vi "3654GetDashValues.vi"   [LabVIEW 2017]
uses:
  <vilib>/Rock Robotics/Network Tables/NT Read Boolean.vi
  Robot Global Data.vi
  <vilib>/Rock Robotics/Network Tables/NT Read Number.vi
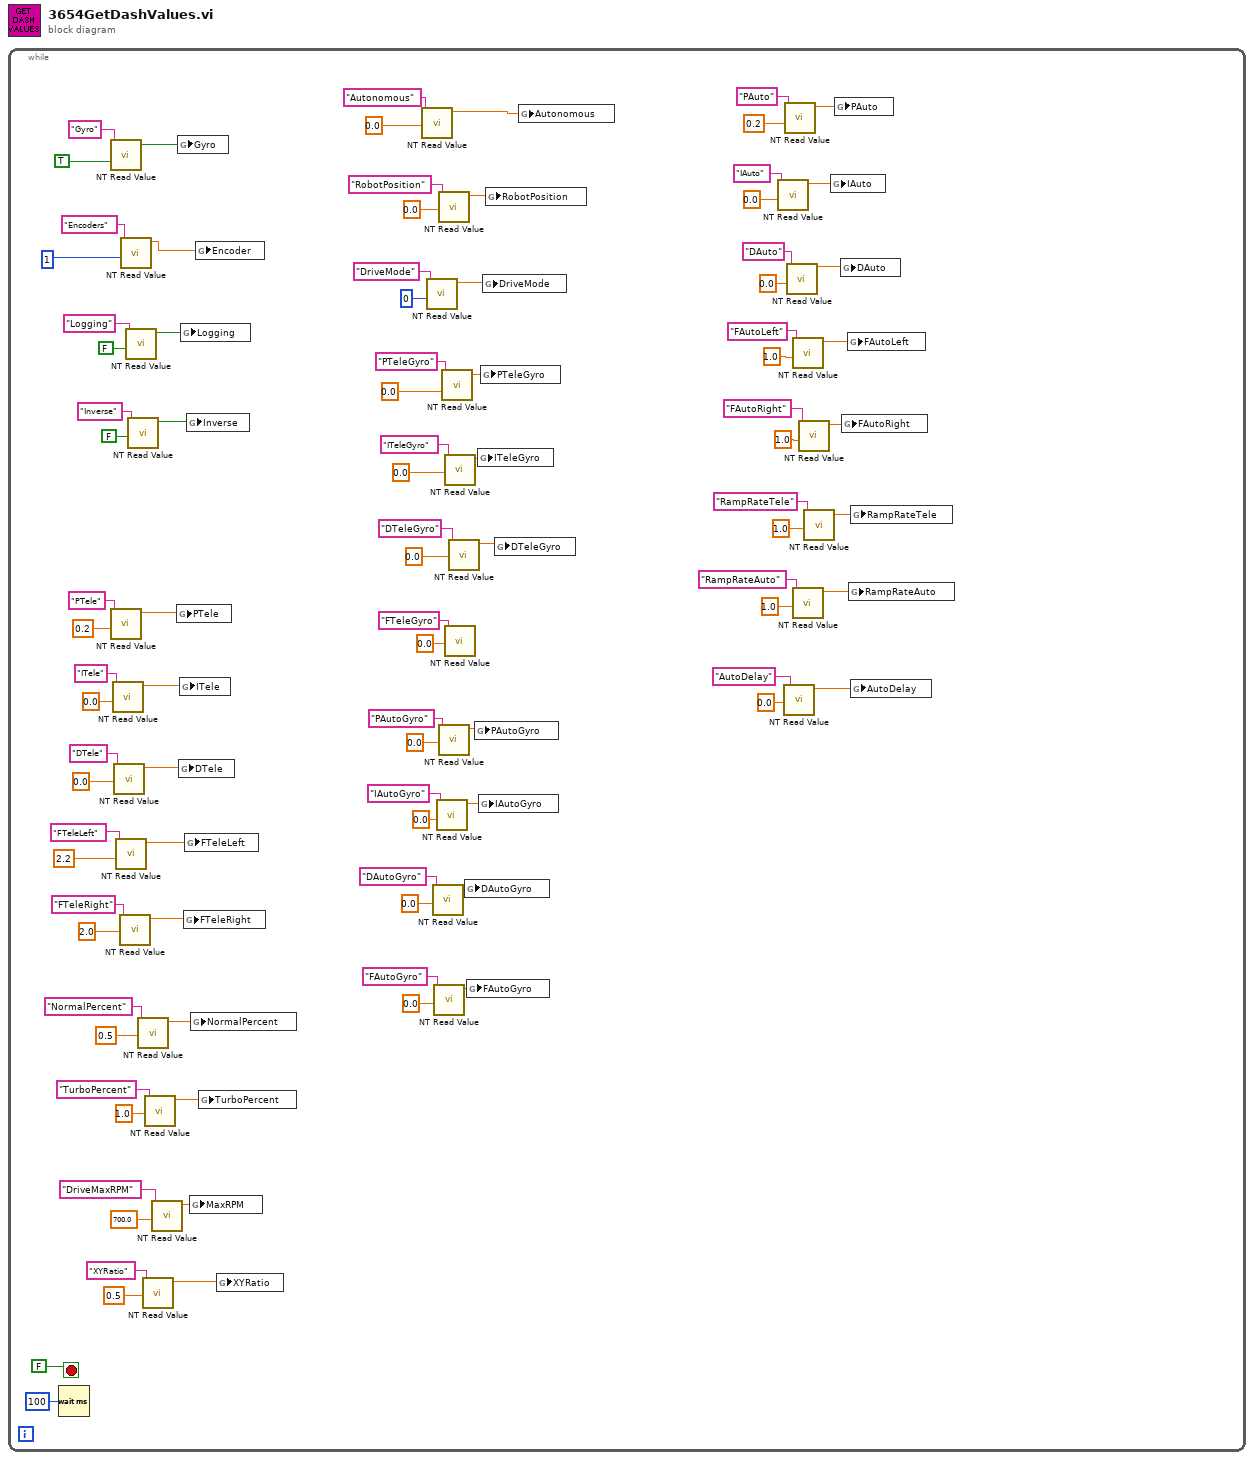
[diagram p0: block diagram]
diagram:
  n1 = while {
    stop <- FALSE stop-if-true
    n2 = Wait (ms)(milliseconds to wait=u32 100) -> ()  [unwired: 1 out]
    n3 = call-poly <vilib>:"NT Read Value.vi"("Default Value"=TRUE, "Name"="Gyro") -> ("Boolean"=w96:bool)  [unwired: 8 in, 1 out]
    n4 = call-poly <vilib>:"NT Read Value.vi"("Default Value"=0.2, "Name"="PTele") -> ("Numeric"=w79:dbl)  [unwired: 8 in, 1 out]
    n5 = call-poly <vilib>:"NT Read Value.vi"("Default Value"=0.0, "Name"="ITele") -> ("Numeric"=w80:dbl)  [unwired: 8 in, 1 out]
    n6 = call-poly <vilib>:"NT Read Value.vi"("Default Value"=0.0, "Name"="DTele") -> ("Numeric"=w81:dbl)  [unwired: 8 in, 1 out]
    n7 = call-poly <vilib>:"NT Read Value.vi"("Default Value"=2.2, "Name"="FTeleLeft") -> ("Numeric"=w72:dbl)  [unwired: 8 in, 1 out]
    n8 = call-poly <vilib>:"NT Read Value.vi"("Default Value"=2.0, "Name"="FTeleRight") -> ("Numeric"=w71:dbl)  [unwired: 8 in, 1 out]
    n9 = call-poly <vilib>:"NT Read Value.vi"("Default Value"=1, "Name"="Encoders") -> ("Numeric"=w2:dbl)  [unwired: 8 in, 1 out]
    n10 = call-poly <vilib>:"NT Read Value.vi"("Default Value"=FALSE, "Name"="Logging") -> ("Boolean"=w31:bool)  [unwired: 8 in, 1 out]
    n11 = call-poly <vilib>:"NT Read Value.vi"("Default Value"=FALSE, "Name"="Inverse") -> ("Boolean"=w32:bool)  [unwired: 8 in, 1 out]
    n12 = call-poly <vilib>:"NT Read Value.vi"("Default Value"=0.5, "Name"="NormalPercent") -> ("Numeric"=w49:dbl)  [unwired: 8 in, 1 out]
    n13 = call-poly <vilib>:"NT Read Value.vi"("Default Value"=0.5, "Name"="XYRatio") -> ("Numeric"=w8:dbl)  [unwired: 8 in, 1 out]
    n14 = call-poly <vilib>:"NT Read Value.vi"("Default Value"=1.0, "Name"="TurboPercent") -> ("Numeric"=w46:dbl)  [unwired: 8 in, 1 out]
    n15 = call-poly <vilib>:"NT Read Value.vi"("Default Value"=700.0, "Name"="DriveMaxRPM") -> ("Numeric"=w11:dbl)  [unwired: 8 in, 1 out]
    n16 = global write "Robot Global Data.vi" "PTele"(w79) -> ()
    n17 = global write "Robot Global Data.vi" "Gyro"(w96) -> ()
    n18 = global write "Robot Global Data.vi" "DTele"(w81) -> ()
    n19 = global write "Robot Global Data.vi" "ITele"(w80) -> ()
    n20 = global write "Robot Global Data.vi" "Logging"(w31) -> ()
    n21 = global write "Robot Global Data.vi" "FTeleRight"(w71) -> ()
    n22 = global write "Robot Global Data.vi" "FTeleLeft"(w72) -> ()
    n23 = global write "Robot Global Data.vi" "Inverse"(w32) -> ()
    n24 = global write "Robot Global Data.vi" "MaxRPM"(w11) -> ()
    n25 = global write "Robot Global Data.vi" "NormalPercent"(w49) -> ()
    n26 = global write "Robot Global Data.vi" "Encoder"(w2) -> ()
    n27 = global write "Robot Global Data.vi" "TurboPercent"(w46) -> ()
    n28 = global write "Robot Global Data.vi" "XYRatio"(w8) -> ()
    n29 = call-poly <vilib>:"NT Read Value.vi"("Default Value"=0.0, "Name"="Autonomous") -> ("Numeric"=w93:dbl)  [unwired: 8 in, 1 out]
    n30 = call-poly <vilib>:"NT Read Value.vi"("Default Value"=0, "Name"="DriveMode") -> ("Numeric"=w5:dbl)  [unwired: 8 in, 1 out]
    n31 = call-poly <vilib>:"NT Read Value.vi"("Default Value"=0.0, "Name"="DAutoGyro") -> ("Numeric"=w41:dbl)  [unwired: 8 in, 1 out]
    n32 = call-poly <vilib>:"NT Read Value.vi"("Default Value"=0.0, "Name"="FAutoGyro") -> ("Numeric"=w20:dbl)  [unwired: 8 in, 1 out]
    n33 = call-poly <vilib>:"NT Read Value.vi"("Default Value"=0.0, "Name"="IAutoGyro") -> ("Numeric"=w42:dbl)  [unwired: 8 in, 1 out]
    n34 = call-poly <vilib>:"NT Read Value.vi"("Default Value"=0.0, "Name"="RobotPosition") -> ("Numeric"=w26:dbl)  [unwired: 8 in, 1 out]
    n35 = call-poly <vilib>:"NT Read Value.vi"("Default Value"=0.0, "Name"="PAutoGyro") -> ("Numeric"=w43:dbl)  [unwired: 8 in, 1 out]
    n36 = call-poly <vilib>:"NT Read Value.vi"("Default Value"=0.0, "Name"="PTeleGyro") -> ("Numeric"=w88:dbl)  [unwired: 8 in, 1 out]
    n37 = call-poly <vilib>:"NT Read Value.vi"("Default Value"=0.0, "Name"="ITeleGyro") -> ("Numeric"=w86:dbl)  [unwired: 8 in, 1 out]
    n38 = call-poly <vilib>:"NT Read Value.vi"("Default Value"=0.0, "Name"="FTeleGyro") -> ()  [unwired: 8 in, 2 out]
    n39 = call-poly <vilib>:"NT Read Value.vi"("Default Value"=0.0, "Name"="DTeleGyro") -> ("Numeric"=w87:dbl)  [unwired: 8 in, 1 out]
    n40 = global write "Robot Global Data.vi" "DAutoGyro"(w41) -> ()
    n41 = global write "Robot Global Data.vi" "FAutoGyro"(w20) -> ()
    n42 = global write "Robot Global Data.vi" "PAutoGyro"(w43) -> ()
    n43 = global write "Robot Global Data.vi" "ITeleGyro"(w86) -> ()
    n44 = global write "Robot Global Data.vi" "IAutoGyro"(w42) -> ()
    n45 = global write "Robot Global Data.vi" "PTeleGyro"(w88) -> ()
    n46 = global write "Robot Global Data.vi" "DriveMode"(w5) -> ()
    n47 = global write "Robot Global Data.vi" "RobotPosition"(w26) -> ()
    n48 = global write "Robot Global Data.vi" "DTeleGyro"(w87) -> ()
    n49 = global write "Robot Global Data.vi" "Autonomous"(w93) -> ()
    n50 = call-poly <vilib>:"NT Read Value.vi"("Default Value"=0.0, "Name"="IAuto") -> ("Numeric"=w63:dbl)  [unwired: 8 in, 1 out]
    n51 = call-poly <vilib>:"NT Read Value.vi"("Default Value"=0.0, "Name"="AutoDelay") -> ("Numeric"=w25:dbl)  [unwired: 8 in, 1 out]
    n52 = call-poly <vilib>:"NT Read Value.vi"("Default Value"=0.2, "Name"="PAuto") -> ("Numeric"=w62:dbl)  [unwired: 8 in, 1 out]
    n53 = call-poly <vilib>:"NT Read Value.vi"("Default Value"=0.0, "Name"="DAuto") -> ("Numeric"=w64:dbl)  [unwired: 8 in, 1 out]
    n54 = call-poly <vilib>:"NT Read Value.vi"("Default Value"=1.0, "Name"="FAutoLeft") -> ("Numeric"=w65:dbl)  [unwired: 8 in, 1 out]
    n55 = call-poly <vilib>:"NT Read Value.vi"("Default Value"=1.0, "Name"="RampRateAuto") -> ("Numeric"=w14:dbl)  [unwired: 8 in, 1 out]
    n56 = call-poly <vilib>:"NT Read Value.vi"("Default Value"=1.0, "Name"="FAutoRight") -> ("Numeric"=w66:dbl)  [unwired: 8 in, 1 out]
    n57 = call-poly <vilib>:"NT Read Value.vi"("Default Value"=1.0, "Name"="RampRateTele") -> ("Numeric"=w17:dbl)  [unwired: 8 in, 1 out]
    n58 = global write "Robot Global Data.vi" "IAuto"(w63) -> ()
    n59 = global write "Robot Global Data.vi" "PAuto"(w62) -> ()
    n60 = global write "Robot Global Data.vi" "DAuto"(w64) -> ()
    n61 = global write "Robot Global Data.vi" "FAutoRight"(w66) -> ()
    n62 = global write "Robot Global Data.vi" "FAutoLeft"(w65) -> ()
    n63 = global write "Robot Global Data.vi" "RampRateAuto"(w14) -> ()
    n64 = global write "Robot Global Data.vi" "RampRateTele"(w17) -> ()
    n65 = global write "Robot Global Data.vi" "AutoDelay"(w25) -> ()
  }
